vi "Autonomous Independent.vi"   [LabVIEW 2015]
doc: "This VI is called when autonomous begins, and will automatically be terminated when autonomous ends. You can carry out timed or sensor driven robot movement independently without needing to return to the caller."
uses:
  <vilib>/Rock Robotics/WPI/Utilities/WPI_GetSetVariantRefNum.vi
  <vilib>/Rock Robotics/WPI/Solenoid/Deprecated/WPI_SolenoidSetBool.vi
panel:
  # "Be sure to right-click and choose Data Operations>>Make Current Value default if you want to save the array values with the VI"
types:
  T1 = typedef "WPI_RobotDriveDevRef.ctl" = cluster{"DevStatus":errorcluster, "Motors[]":T2[], "Square Inputs":bool, "Max Output":dbl}
  T2 = typedef "WPI_MotorControlDeviceRef.ctl" = cluster{"DeviceStatus":errorcluster, "Type":T3, "PWM":cluster{"PWM Channel":T4, "DeadBand":T5}, "CAN":cluster{"Device Number":u8, "Control Mode":T6, "Semaphore":T7, "Max Vout":dbl, "TalonSRX Control Mode":T8}, "Invert":bool}
  T3 = typedef "WPI_MotorControlType.ctl" = enum16{"PWM", "CAN", "CANTalonSRX"}
  T4 = typedef "FPGA_DIOPWMChannel.ctl" = enum8{"PWM 0", "PWM 1", "PWM 2", "PWM 3", "PWM 4", "PWM 5", "PWM 6", "PWM 7", "PWM 8", "PWM 9", "PWM MXP 0", "PWM MXP 1", "PWM MXP 2", "PWM MXP 3", "PWM MXP 4", "PWM MXP 5", "PWM MXP 6", "PWM MXP 7", "PWM MXP 8", "PWM MXP 9", "Invalid"}
  T5 = typedef "WPI_PWMDeadband.ctl" = cluster{"Name":string, "maxPositivePwm":i32, "minPositivePwm":i32, "centerPwm":i32, "maxNegativePwm":i32, "minNegativePwm":i32, "angularRange":u16}
  T6 = typedef "WPI_CANJaguar_ControlMode.ctl" = enum8{"Percent VBus", "Current", "Speed", "Position", "Voltage"}
  T7 = typedef "Semaphore RefNum" = refnum<k1>
  T8 = typedef "WPI_CANTalonSRX_APIControlMode.ctl" = enum8{"Percent VBus", "Speed", "Position", "Slave", "Unchanged / Invalid", "Voltage Compensation", "Current", "Motion Profile"}
  T9 = typedef "WPI_SolenoidDevRef.ctl" = cluster{"DevStatus":errorcluster, "Pneumatics Control Module":u8, "Forward Solenoid Channel":T10, "Reverse Solenoid Channel":T10}
  T10 = typedef "WPI_SolenoidChannel.ctl" = enum8{"Solenoid 0", "Solenoid 1", "Solenoid 2", "Solenoid 3", "Solenoid 4", "Solenoid 5", "Solenoid 6", "Solenoid 7", "Invalid"}
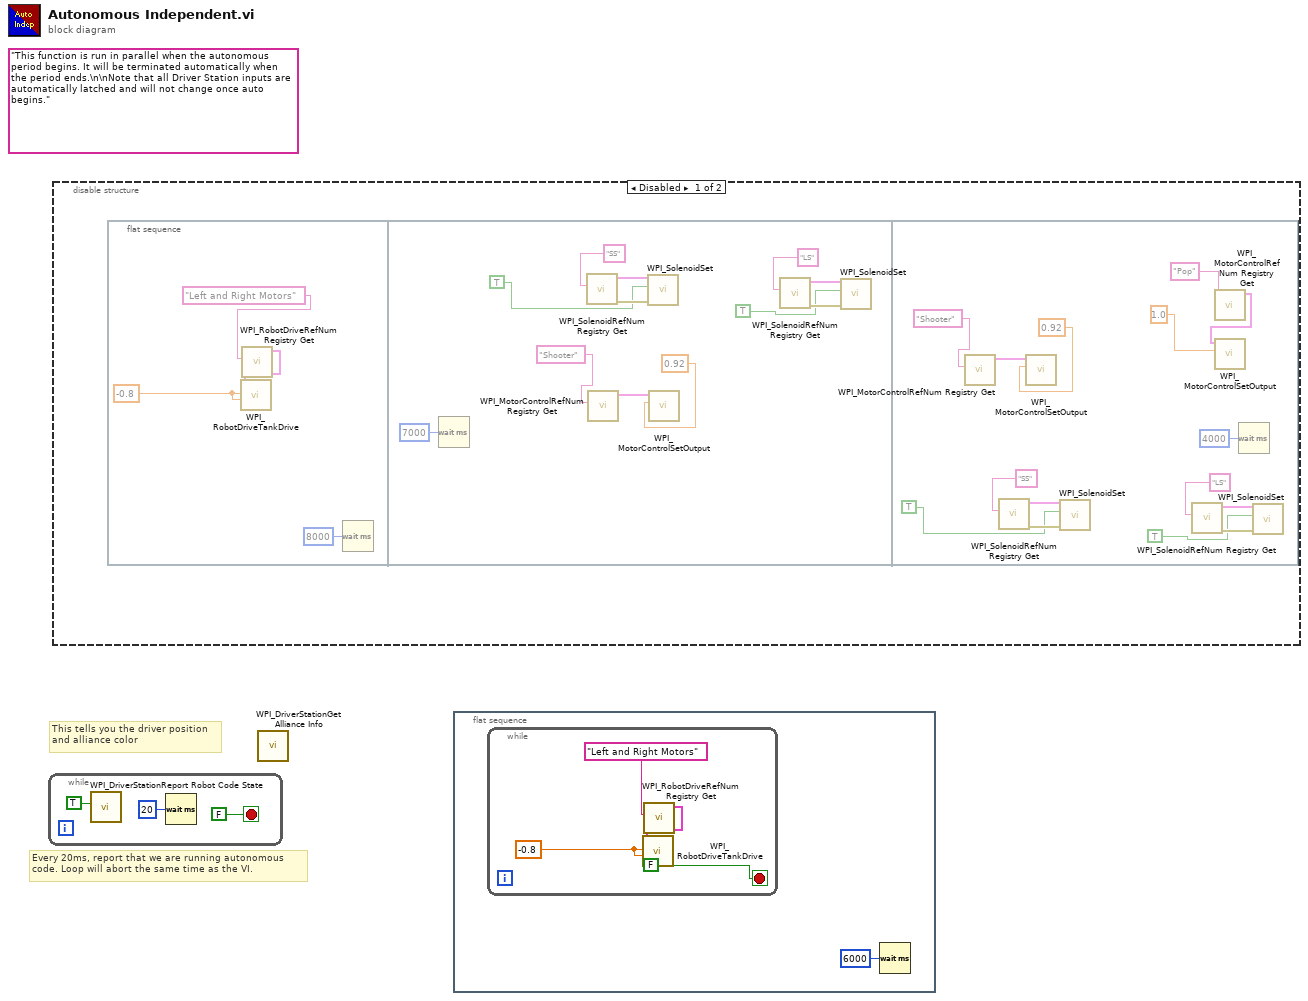
[diagram p0: block diagram]
diagram:
  (unwired) "This function is run in parallel when the autonomous period begins. It will be terminated automatically when the period ends.\n\nNote that all Driver Station inputs are automatically latched and will not change once auto begins."
  # "Every 20ms, report that we are running autonomous\ncode. Loop will abort the same time as the VI."
  # "This tells you the driver position\nand alliance color"
  n1 = while {
    stop <- FALSE stop-if-true
    n2 = call <vilib>:"WPI_DriverStationReport Robot Code State.vi"("Autonomous"=TRUE) -> ()  [unwired: 10 in, 1 out]
    n3 = Wait (ms)(milliseconds to wait=u32 20) -> ()  [unwired: 1 out]
  }
  n4 = disable-structure shown="Disabled" {
    frame Disabled {
      n5 = flat-sequence {
        frame #0 {
          w4 = -0.8
          n6 = call <vilib>:"WPI_RobotDriveRefNum Registry Get.vi"("refnum name"="Left and Right Motors") -> ("RobotDriveDevRef"=w5:T1)  [unwired: 9 in, 1 out]
          n7 = call <vilib>:"WPI_RobotDriveTankDrive.vi"("Right axis value"=w4, "Left axis value"=w4, "RobotDriveDevRef"=w5) -> ()  [unwired: 6 in, 3 out]
          n8 = Wait (ms)(milliseconds to wait=u32 8000) -> ()  [unwired: 1 out]
        }
        frame #1 {
          n9 = Wait (ms)(milliseconds to wait=u32 7000) -> ()  [unwired: 1 out]
          n10 = call <vilib>:"WPI_SolenoidRefNum Registry Get.vi"("refnum name"="SS") -> ("error out"=w14:errorcluster, "SolenoidDevRef"=w15:T9)  [unwired: 9 in]
          n11 = call <vilib>:"WPI_MotorControlRefNum Registry Get.vi"("refnum name"="Shooter") -> ("MotorControlDevRef"=w19:T2)  [unwired: 9 in, 1 out]
          n12 = call-poly <vilib>:"WPI_SolenoidSet.vi"("error in (no error)"=w14, "Value"=TRUE, "SolenoidDevRef"=w15) -> ()  [unwired: 9 out]
          n13 = call <vilib>:"WPI_MotorControlSetOutput.vi"("Output"=0.92, "MotorControlDevRef"=w19) -> ()  [unwired: 7 in, 3 out]
          n14 = call <vilib>:"WPI_SolenoidRefNum Registry Get.vi"("refnum name"="LS") -> ("error out"=w11:errorcluster, "SolenoidDevRef"=w12:T9)  [unwired: 9 in]
          n15 = call-poly <vilib>:"WPI_SolenoidSet.vi"("error in (no error)"=w11, "Value"=TRUE, "SolenoidDevRef"=w12) -> ()  [unwired: 9 out]
        }
        frame #2 {
          n16 = call <vilib>:"WPI_MotorControlRefNum Registry Get.vi"("refnum name"="Shooter") -> ("MotorControlDevRef"=w31:T2)  [unwired: 9 in, 1 out]
          n17 = call <vilib>:"WPI_SolenoidRefNum Registry Get.vi"("refnum name"="SS") -> ("error out"=w26:errorcluster, "SolenoidDevRef"=w27:T9)  [unwired: 9 in]
          n18 = call <vilib>:"WPI_MotorControlSetOutput.vi"("Output"=0.92, "MotorControlDevRef"=w31) -> ()  [unwired: 7 in, 3 out]
          n19 = call-poly <vilib>:"WPI_SolenoidSet.vi"("error in (no error)"=w26, "Value"=TRUE, "SolenoidDevRef"=w27) -> ()  [unwired: 9 out]
          n20 = call <vilib>:"WPI_SolenoidRefNum Registry Get.vi"("refnum name"="LS") -> ("error out"=w23:errorcluster, "SolenoidDevRef"=w24:T9)  [unwired: 9 in]
          n21 = call <vilib>:"WPI_MotorControlRefNum Registry Get.vi"("refnum name"="Pop") -> ("MotorControlDevRef"=w33:T2)  [unwired: 9 in, 1 out]
          n22 = call <vilib>:"WPI_MotorControlSetOutput.vi"("Output"=1.0, "MotorControlDevRef"=w33) -> ()  [unwired: 7 in, 3 out]
          n23 = Wait (ms)(milliseconds to wait=u32 4000) -> ()  [unwired: 1 out]
          n24 = call-poly <vilib>:"WPI_SolenoidSet.vi"("error in (no error)"=w23, "Value"=TRUE, "SolenoidDevRef"=w24) -> ()  [unwired: 9 out]
        }
      }
    }
    frame Enabled {
    }
  }
  n25 = call <vilib>:"WPI_DriverStationGet Alliance Info.vi"() -> ()  [unwired: 12 out]
  n26 = flat-sequence {
    frame #0 {
      n27 = while {
        stop <- FALSE stop-if-true
        w37 = -0.8
        n28 = call <vilib>:"WPI_RobotDriveRefNum Registry Get.vi"("refnum name"="Left and Right Motors") -> ("RobotDriveDevRef"=w38:T1)  [unwired: 9 in, 1 out]
        n29 = call <vilib>:"WPI_RobotDriveTankDrive.vi"("Right axis value"=w37, "Left axis value"=w37, "RobotDriveDevRef"=w38) -> ()  [unwired: 6 in, 3 out]
      }
      n30 = Wait (ms)(milliseconds to wait=u32 6000) -> ()  [unwired: 1 out]
    }
  }
